vi "Loop Async.vi"(4 "MultiErrors":refnum<class "MultiErrors.lvclass">, 5 "Sequencer":refnum<class "MessageQ.lvclass">, 6 "Sequence Control":T1, 7 "VolatusAPI":refnum<class "VolatusAPI.lvclass">, 9 "Promise":refnum<class "Promise.lvclass">, 10 "State":T2, 11 "State in":refnum<class "State.lvclass">) -> ()   [LabVIEW 2023, in "VolatusSeq.lvlib" / "State.lvclass"]
uses:
  State.lvclass
  lv-promises/Promises/Promise/Promise.lvclass
  VolatusSeqConfig/State.ctl
  VolatusSeqConfig/Step.ctl
  Volatus/VolatusAPI/VolatusAPI.lvclass
  State Control.ctl
  Sequence Time.ctl
  Variables/Variables.lvclass
  VolatusErrorUtilities/MultiErrors/MultiErrors.lvclass
  Volatus/MessageQ/MessageQ.lvclass
  lv-promises/Promises/Value/Value.lvclass
  VolatusErrorUtilities/MultiErrors/MultiErrors.lvclass/MultiErrors.ctl
  State.lvclass/State.ctl
  VolatusSeqConfig/Command Config/Command Config.lvclass
  VolatusSeqConfig/VolatusSeqConfig.lvlib
  VolatusSeqConfig/Transition Config/Transition Config.lvclass
  VolatusSeq.lvlib
  VolatusSeqConfig/Debug Flags.ctl
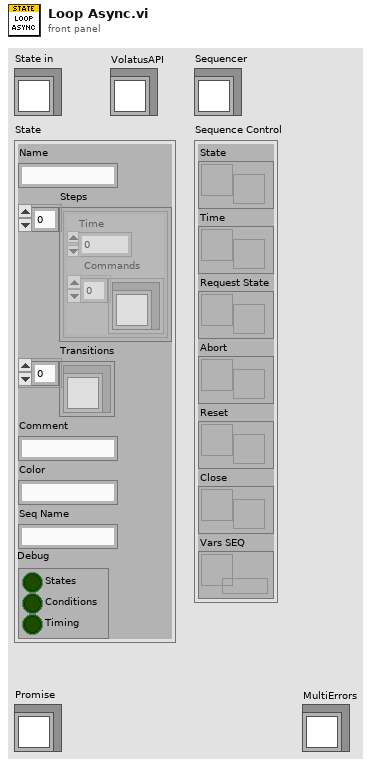
[diagram p1: front panel]
types:
  T1 = typedef "VolatusSeq.lvlib/State Control.ctl" = cluster{"State":refnum<notifier>, "Time":refnum<notifier>, "Request State":refnum<notifier>, "Abort":refnum<notifier>, "Reset":refnum<notifier>, "Close":refnum<notifier>, "Vars SEQ":refnum<queue>}
  T2 = typedef "VolatusSeqConfig.lvlib/State.ctl" = cluster{"Name":string, "Steps":T3[], "Transitions":refnum<class "Transition Config.lvclass">[], "Comment":string, "Color":string, "Seq Name":string, "Debug":T4}
  T3 = typedef "VolatusSeqConfig.lvlib/Step.ctl" = cluster{"Time":dbl, "Commands":refnum<class "Command Config.lvclass">[]}
  T4 = typedef "VolatusSeqConfig.lvlib/Debug Flags.ctl" = cluster{"States":bool, "Conditions":bool, "Timing":bool}
  T5 = typedef "VolatusSeq.lvlib/State.lvclass/State Loop Data.ctl" = cluster{"Next Index":i32, "Step Time":dbl[], "Step Commands":cluster{"Commands":T6[]}[], "Transitions":refnum<class "Transition.lvclass">[], "Time":T11, "Actions":refnum<class "Iteration Actions.lvclass">[], "Variables":refnum<class "Variables.lvclass">, "Action":refnum<class "Iteration Actions.lvclass">, "Debug":T4}
  T6 = typedef "VolatusSeq.lvlib/Command.ctl" = cluster{"Type":T7, "MsgQ":refnum<class "MessageQ.lvclass">, "Strings":string[], "CmdDigital":T8, "CmdAnalog":T9, "Send Type":T10, "Node":string, "Task":string, "I32s":i32[], "Channel DBLs":refnum<class "Channel DBL.lvclass">[], "F String":refnum<class "Format String.lvclass">}
  T7 = typedef "VolatusSeqConfig.lvlib/Command Type.ctl" = enum16{"Digital", "Numeric", "Transition", "Stop", "StartLog", "StopLog", "Start", "Event", "Error", "HTTP", "ResetVar", "IncVar", "DecVar", "SaveVar", "LoadVar", "AddVar", "SubVar", "SetVar", "AddToVar"}
  T8 = typedef "CmdDigital.lvlib/Data.ctl" = cluster{"channel":string, "value":bool}
  T9 = typedef "CmdAnalog.lvlib/Data.ctl" = cluster{"channel":string, "value":dbl}
  T10 = typedef "VolatusSeq.lvlib/Send Type.ctl" = enum16{"Local", "Remote"}
  T11 = typedef "VolatusSeq.lvlib/Sequence Time.ctl" = cluster{"Abort":bool, "Seq Time":dbl, "State Time":dbl, "Wall Time":dbl}
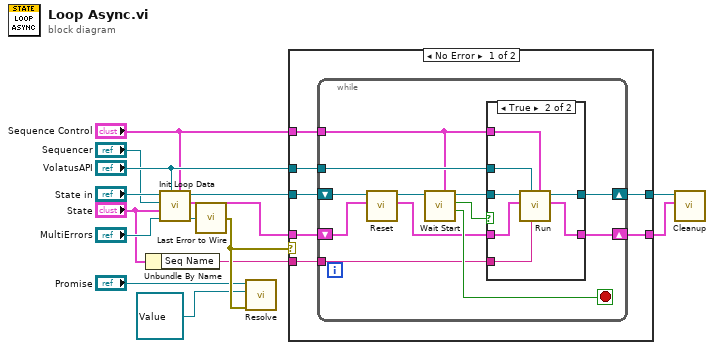
[diagram p0: block diagram]
diagram:
  n1 = Unbundle By Name("State") -> ("Seq Name"=w5:string)
  n2 = call "Init Loop Data.vi"("State Control"="Sequence Control", "VolatusAPI"="VolatusAPI", "MultiErrors"="MultiErrors", "State"="State", "Sequencer"="Sequencer", "State in"="State in") -> ("error out"=w6:refnum<class "MultiErrors.lvclass">, "State Loop Data"=w12:T5, "State out"=w10:refnum<class "State.lvclass">)  [unwired: 3 in]
  n3 = call "Last Error to Wire.vi"("MultiErrors in"=w6) -> ("error out"=w15:errorcluster)  [unwired: 8 in]
  n4 = call "Resolve.vi"("error in (no error)"=w15, "Result (None)"=refnum<class "Value.lvclass"> refnum ("Result"), "Promise in"="Promise") -> ()  [unwired: 7 in, 2 out]
  n5 = case shown="No Error" w15 {
    tunnel: w12 -> [w22 w44]
    tunnel: "VolatusAPI" -> [w21 _]
    tunnel: w10 -> [w20 w45]
    tunnel: [w19 w45] -> w9
    tunnel: "Sequence Control" -> [w18 _]
    tunnel: w5 -> [w17 _]
    tunnel: [w16 w44] -> w1
    frame No Error {
      n6 = while {
        shift-right: [w29] -> w16
        shift-left: w22 -> [w27]
        tunnel: w21 -> [w31]
        shift-right: [w30] -> w19
        shift-left: w20 -> [w28]
        tunnel: w18 -> [w24]
        tunnel: w17 -> [w23]
        stop <- w33 stop-if-true
        n7 = call "Reset.vi"("State Loop Data in"=w27, "State in"=w28) -> ("State Loop Data"=w25:T5, "State out"=w26:refnum<class "State.lvclass">)  [unwired: 8 in]
        n8 = call "Wait Start.vi"("Sequence Control"=w24, "State in"=w26) -> ("Close"=w33:bool, "Start"=w34:bool, "State out"=w32:refnum<class "State.lvclass">)  [unwired: 6 in, 1 out]
        n9 = case shown="True" w34 {
          tunnel: w32 -> [w36 w39]
          tunnel: w31 -> [_ w42]
          tunnel: w25 -> [w35 w40]
          tunnel: [w36 w43] -> w30
          tunnel: [w35 w41] -> w29
          tunnel: w24 -> [_ w38]
          tunnel: w23 -> [_ w37]
          frame False {
          }
          frame True {
            n10 = call "Run.vi"("Sequence Control"=w38, "Seq Name"=w37, "VolatusAPI"=w42, "State Loop Data in"=w40, "State in"=w39) -> ("State Loop Data"=w41:T5, "State out"=w43:refnum<class "State.lvclass">)  [unwired: 5 in]
          }
        }
      }
    }
    frame Error {
    }
  }
  n11 = call "Cleanup.vi"("State Loop Data"=w1, "State in"=w9) -> ()  [unwired: 9 in, 1 out]
